vi "SHA-1 (File).vi"(10 "filepath":path) -> (2 "SHA-1 hash":string)   [LabVIEW 2013, in "SHA-1.lvlib"]
uses:
  SHA-1.lvlib
  class/SHA-1.lvclass
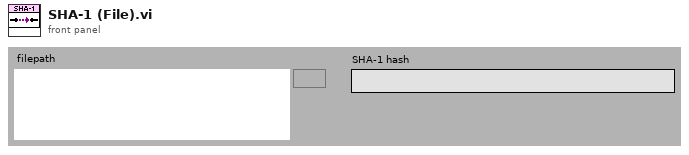
[diagram p1: front panel]
types:
  T1 = enum16{"open", "replace", "create", "open or create", "replace or create", "replace or create with confirmation"}
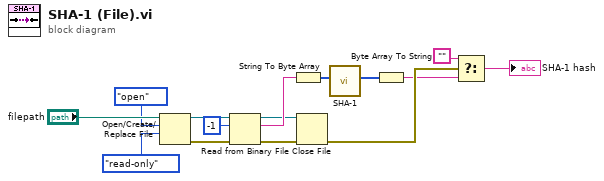
[diagram p0: block diagram]
diagram:
  n1 = Open/Create/Replace File(file path (use dialog)="filepath", operation (0:open)=T1."open", access (0:read/write)=enum16{"read/write", "read-only", "write-only"}."read-only") -> (refnum out=w9:refnum<file>, error out=w1:errorcluster)  [unwired: 3 in, 1 out]
  n2 = Read from Binary File(8:w1, 10:-1 ("count (1)"), 11:w9) -> (0:w2:errorcluster, 2:w8:string, 3:w6:refnum<file>)  [unwired: 3 in, 1 out]
  n3 = String To Byte Array(string=w8) -> (unsigned byte array=w14:u8[])
  n4 = Close File(refnum=w6, error in=w2) -> (error out=w5:errorcluster)  [unwired: 1 out]
  n5 = call "SHA-1.vi"("data"=w14) -> ("SHA-1 hash"=w15:u8[])  [unwired: 10 in]
  n6 = Byte Array To String(unsigned byte array=w15) -> (string=w4:string)
  n7 = Select(t="", s=w5, f=w4) -> (s? t:f=→"SHA-1 hash":string)
